vi "Test Paths.vi"(10 "Test Type":T1) -> (2 "Path":path)   [LabVIEW 2020, in "UT_CICD.lvlib"]
uses:
  UT_CICD.lvlib
  Test Types--enum.ctl
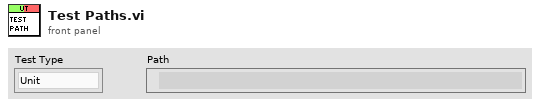
[diagram p1: front panel]
types:
  T1 = typedef "UT_CICD.lvlib/Test Types--enum.ctl" = enum16{"Unit", "Integration", "E2E"}
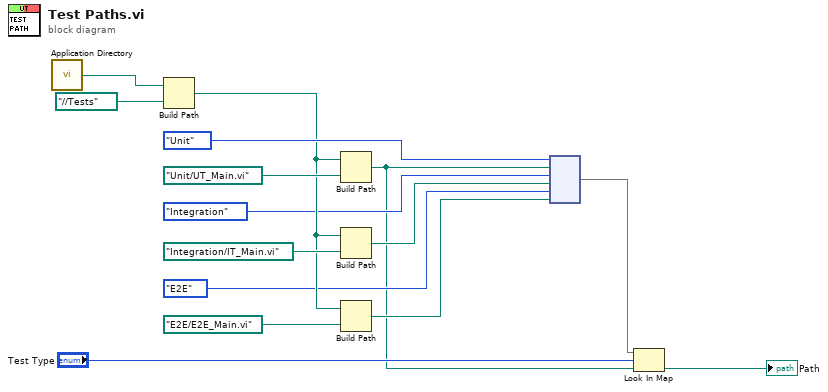
[diagram p0: block diagram]
diagram:
  n1 = call <vilib>:"Application Directory.vi"() -> ("Application Directory"=w15:path)
  n2 = Build Path(base path=w15, name or relative path=path "../../Tests") -> (appended path=w7:path)
  n3 = Build Path(base path=w7, name or relative path=path "Unit/UT_Main.vi") -> (appended path=w2:path)
  n4 = Build Path(base path=w7, name or relative path=path "Integration/IT_Main.vi") -> (appended path=w9:path)
  n5 = Build Path(base path=w7, name or relative path=path "E2E/E2E_Main.vi") -> (appended path=w8:path)
  n6 = node(Test_Types--enum."Unit", w2, Test_Types--enum."Integration", w9, Test_Types--enum."E2E", w8) -> (w4:map{T1, path})
  n7 = Look In Map(map=w4, key="Test Type", default value=w2) -> (value=→"Path":path)  [unwired: 1 out]
